vi "clear Port.vi"(11 "port_num":i32) -> ()   [LabVIEW 2016, in "dxl_x86_c.lvlib"]
doc: "WINDECLSPEC void clearPort (int port_num);"
uses:
  dxl_x86_c.lvlib
  dxl_x86_c.dll
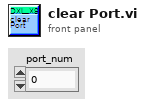
[diagram p1: front panel]
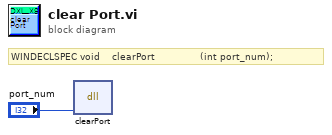
[diagram p0: block diagram]
diagram:
  # "WINDECLSPEC void    clearPort               (int port_num);"
  n1 = dll-call lib="C:/Users/Platform/Desktop/DynamixelSDK/labview/dxl_x86_c.lvlib/dxl_x86_c.*" fn="clearPort"("port_num"="port_num") -> ()  [unwired: 5 in, 2 out]
